vi "Capture@ROITranslate__Parameter.vi"(1 "ParamterIn":string) -> (0 "ParamterOut":string)   [LabVIEW 2019]
panel:
  in  "YEdge":string(combo)
  in  "XEdge":string(combo)
  in  "CamName":string(combo)
  in  "Confirm":bool
  # "Capture@ROITranslate $Capture,$Base,$New\n -----> $Base=[X,Y,0,U]\n             $New=[X',Y',0,U']"
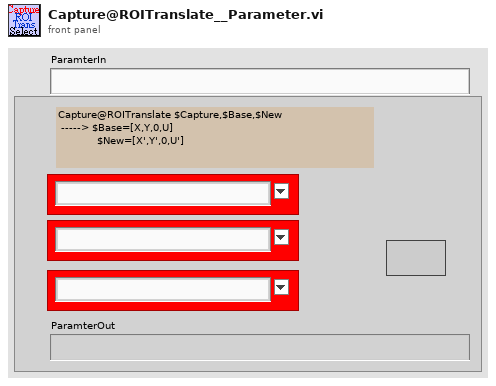
[diagram p1: front panel]
types:
  T1 = enum16{"Get", "UpdatePointS", "Init", "UpdateIndex", "GetCurrent&Index+1", "GetWithIndex", "ChkLast", "GetCurrent"}
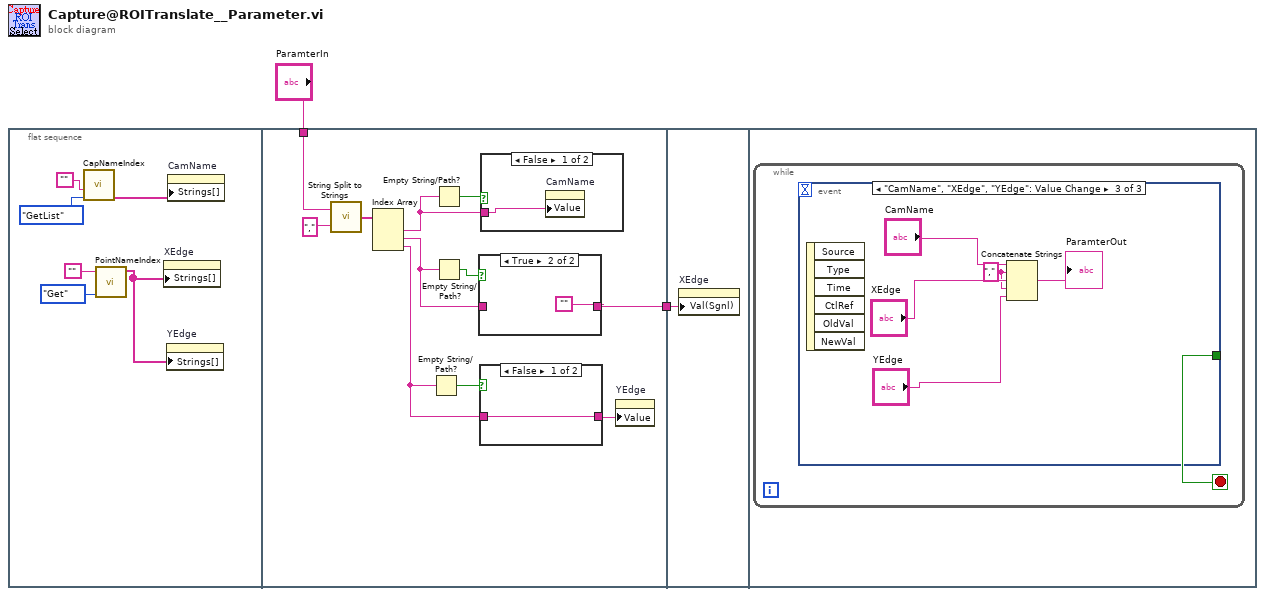
[diagram p0: block diagram]
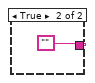
[diagram p2: hidden frame]
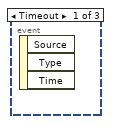
[diagram p5: hidden frame]
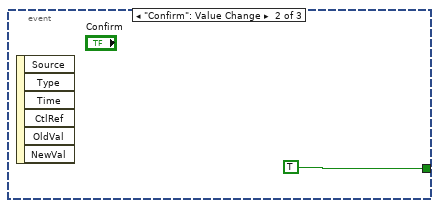
[diagram p6: hidden frame]
diagram:
  n1 = flat-sequence {
    tunnel: "ParamterIn" -> [w17]
    tunnel: [w12] -> w1
    tunnel: w1 -> [w25]
    frame #0 {
      n2 = call "CapNameIndex.vi"("OP"=enum16{"AddCam", "GetIndex", "Init", "GetList"}."GetList", "CamName"="") -> ("DeviceList"=w7:string[])  [unwired: 2 in, 3 out]
      n3 = call "PointNameIndex.vi"("OP"=T1."Get", "PointName"="") -> ("PointNameList"=w3:string[])  [unwired: 4 in, 5 out]
      n4 = property on="XEdge" class="CmbBox"("Strings[]"=w3) -> ()  [unwired: 2 in, 2 out]
      n5 = property on="YEdge" class="CmbBox"("Strings[]"=w3) -> ()  [unwired: 2 in, 2 out]
      n6 = property on="CamName" class="CmbBox"("Strings[]"=w7) -> ()  [unwired: 2 in, 2 out]
    }
    frame #1 {
      n7 = call "String Split to Strings.vi"("search string/char (-)"=",", "String"=w17) -> ("Array"=w19:string[])
      n8 = Index Array(array=w19) -> (element #1=w15:string, element #2=w13:string, element #3=w10:string)  [unwired: 3 in]
      n9 = Empty String/Path?(string/path=w10) -> (empty?=w11:bool)
      n10 = Empty String/Path?(string/path=w15) -> (empty?=w16:bool)
      n11 = Empty String/Path?(string/path=w13) -> (empty?=w14:bool)
      n12 = case shown="True" w14 {
        tunnel: [w22 ""] -> w12
        tunnel: w13 -> [w22 _]
        frame False {
        }
        frame True {
        }
      }
      n13 = case shown="False" w11 {
        tunnel: [w20 ""] -> w9
        tunnel: w10 -> [w20 _]
        frame False {
        }
        frame True {
        }
      }
      n14 = case shown="False" w16 {
        tunnel: w15 -> [w24 _]
        frame False {
          n15 = property on="CamName" class="CmbBox"("Value"=w24) -> ()  [unwired: 2 in, 2 out]
        }
        frame True {
        }
      }
      n16 = property on="YEdge" class="CmbBox"("Value"=w9) -> ()  [unwired: 2 in, 2 out]
    }
    frame #2 {
      n17 = property on="XEdge" class="CmbBox"("Val(Sgnl)"=w25) -> ()  [unwired: 2 in, 2 out]
    }
    frame #3 {
      n18 = while {
        stop <- w26 stop-if-true
        n19 = event shown="[2] \"CamName\", \"XEdge\", \"YEdge\": Value Change" {
          selector: _ -> [_ _ _]
          dyn-events: _ -> [_ _ _]
          timeout: _ -> [_ _ _]
          tunnel: [_ TRUE _] -> w26
          event Timeout {
            n20 = event-data() -> ()  [unwired: 1 in, 3 out]
          }
          event "Confirm": Value Change {
            n21 = event-data() -> ()  [unwired: 1 in, 6 out]
          }
          event "CamName", "XEdge", "YEdge": Value Change {
            w29 = "," ("string")
            n22 = event-data() -> ()  [unwired: 1 in, 6 out]
            n23 = Concatenate Strings("CamName", w29, "XEdge", w29, "YEdge") -> (→"ParamterOut":string)
          }
        }
      }
    }
  }
